vi "Get_ini_Reference.vi"(6 "create file if necessary? (T)":bool=TRUE, 7 "Ignore Errors (F)":bool, 8 "Error in":errorcluster, 10 "ini file name":string) -> (0 "Error out":errorcluster, 3 "ini Ref":T1, 5 "ini file path":path)   [LabVIEW 2011]
doc: "Get ini Reference\nver. 1.3 - Feb. 2004\nAuthor - Ed Dickens - edwind@distek.com\n\nThis VI will open a reference to the specified ini file assuming it is in the same folder as the top level VI, LLB or exe. If the \"ini file name\" control is left empty, this VI will get the name of the calling VI and use that to build the ini file name. It also will remove any name-mangled/namespace suffixes before building the name.\n\nExamples:\nSub-VI1.vi = Sub-VI1.ini\nSub-VI2__ogtk.vi = Sub-VI2.ini"
uses:
  <vilib>/Utility/config.llb/Config Data RefNum.ctl
  libs/File/Strip Path Extension - String__ogtk.vi
  <vilib>/Utility/config.llb/NI_LVConfig.lvlib
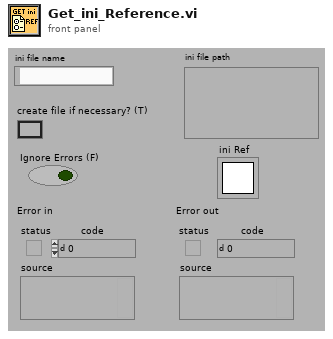
[diagram p1: front panel]
types:
  T1 = typedef "NI_LVConfig.lvlib/Config Data RefNum.ctl" = refnum<k1>
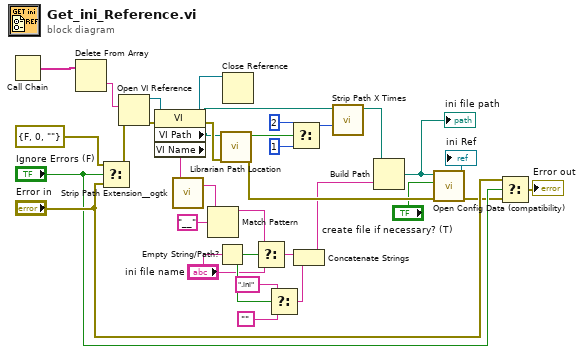
[diagram p0: block diagram]
diagram:
  n1 = Call Chain() -> (call chain=w2:string[])
  n2 = Delete From Array(array=w2) -> (deleted portion=w1:string)  [unwired: 2 in, 1 out]
  n3 = Select(t=errorcluster {"status"=FALSE, "code"=0, "source"=""}, s="Ignore Errors (F)", f="Error in") -> (s? t:f=w8:errorcluster)
  n4 = Open VI Reference(vi path=w1, error in (no error)=w8) -> (vi reference=w29:refnum<vi>, error out=w30:errorcluster)  [unwired: 4 in]
  n5 = property class="VI"(reference=w29, error in=w30) -> (reference out=w27:refnum<vi>, error out=w28:errorcluster, "VI Path"=w14:path, "VI Name"=w17:string)
  n6 = call-poly "Strip Path Extension__ogtk.vi"("path"=w17) -> ("root"=w16:string)  [unwired: 1 out]
  n7 = Match Pattern(string=w16, regular expression="__") -> (before substring=w15:string)  [unwired: 1 in, 3 out]
  n8 = Empty String/Path?(string/path="ini file name") -> (empty?=w25:bool)
  n9 = call <vilib>:"Librarian Path Location.vi"("error in (no error)"=w28, "path"=w14) -> ("error out"=w33:errorcluster, "path is in a VI library"=w12:bool)  [unwired: 5 in, 3 out]
  n10 = Close Reference(reference=w27) -> ()  [unwired: 1 in, 1 out]
  n11 = Select(t=w15, s=w25, f="ini file name") -> (s? t:f=w24:string)
  n12 = Select(t=".ini" ("Substring"), s=w25, f="") -> (s? t:f=w22:string)
  n13 = Select(t=2 ("# to Strip(2)"), s=w12, f=1 ("# to Strip(2)")) -> (s? t:f=w9:i32)
  n14 = Concatenate Strings(w24, w22) -> (w23:string)
  n15 = call "Strip Path X Times.vi"("# to Strip(2)"=w9, "Path"=w14) -> ("Stripped Path"=w13:path)  [unwired: 8 in, 1 out]
  n16 = Build Path(base path=w13, name or relative path=w23) -> (appended path=w32:path)
  "ini file path" <- w32
  n17 = call <vilib>:"Open Config Data (compatibility).vi"("error in (no error)"=w33, "create file if necessary (T)"="create file if necessary? (T)", "configuration file path"=w32) -> ("error out"=w3:errorcluster, "refnum"=→"ini Ref":T1)  [unwired: 6 in, 1 out]
  n18 = Select(t="Error in", s="Ignore Errors (F)", f=w3) -> (s? t:f=→"Error out":errorcluster)
